vi "log_error.vi"(6 "timestamp":timestamp, 7 "context":string, 8 "error in (no error)":errorcluster, 9 "level":T1=200 items=["OFF"=0, "FATAL"=100, "ERROR"=200, "WARN"=300, "INFO"=400, "DEBUG"=500, "TRACE"=600, "ALL"=65535], 11 "Queue Log Provider in":refnum<class "NIErrLog Log Provider.lvclass">) -> (0 "error out":errorcluster, 3 "Queue Log Provider out":refnum<class "NIErrLog Log Provider.lvclass">)   [LabVIEW 2019, in "LVCOOOP.lvlib" / "Support API.lvlib" / "NIErrLog Log Provider.lvclass"]
uses:
  NIErrLog Log Provider.lvclass
  Log Service/public/level.ctl
  Log Service/Log Service.lvclass
  <vilib>/Utility/SystemLogging/NI_SystemLogging.lvlib
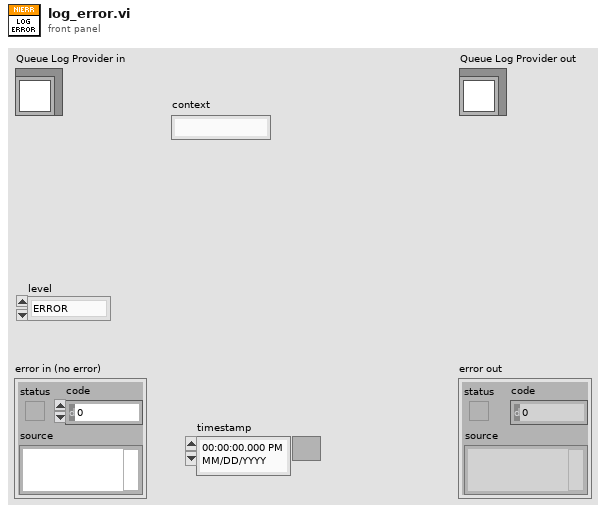
[diagram p1: front panel]
types:
  T1 = typedef "LVCOOOP.lvlib/Support API.lvlib/Log Service.lvclass/level.ctl" = u16
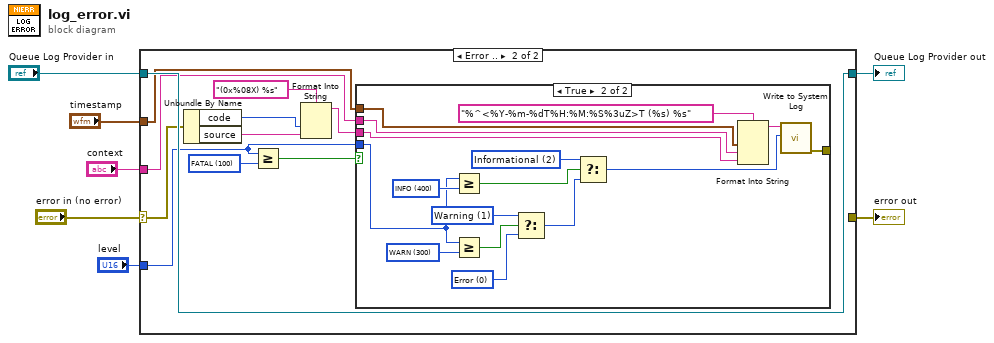
[diagram p0: block diagram]
diagram:
  n1 = case shown="Error .." "error in (no error)" {
    selector: "error in (no error)" -> [w9 w19]
    tunnel: [w9 _] -> w1
    tunnel: "timestamp" -> [_ w13]
    tunnel: "level" -> [_ w10]
    tunnel: "context" -> [_ w12]
    tunnel: [w8 w20] -> w5
    tunnel: "Queue Log Provider in" -> [w8 w20]
    frame No Error {
    }
    frame Error {
      w15 = T1 100 items=["OFF"=0, "FATAL"=100, "ERROR"=200, "WARN"=300, "INFO"=400, "DEBUG"=500, "TRACE"=600, "ALL"=65535] ("level")
      n2 = Unbundle By Name(w19) -> ("code"=w17:i32, "source"=w16:string)
      n3 = Greater Or Equal?(x=w10, y=w15) -> (x >= y?=w14:bool)
      n4 = Format Into String(format string="(0x%08X) %s", w17, w16) -> (resulting string=w11:string)  [unwired: 2 in, 1 out]
      n5 = case shown="True" w14 {
        tunnel: w10 -> [_ w29]
        tunnel: [_ w26] -> _
        tunnel: w11 -> [_ w21]
        tunnel: w12 -> [_ w22]
        tunnel: w13 -> [_ w23]
        frame False {
        }
        frame True {
          w28 = 0 items=["Error", "Warning", "Informational"] ("severity")
          w31 = 1 items=["Error", "Warning", "Informational"] ("severity")
          w33 = T1 300 items=["OFF"=0, "FATAL"=100, "ERROR"=200, "WARN"=300, "INFO"=400, "DEBUG"=500, "TRACE"=600, "ALL"=65535] ("level")
          w34 = 2 items=["Error", "Warning", "Informational"] ("severity")
          w36 = T1 400 items=["OFF"=0, "FATAL"=100, "ERROR"=200, "WARN"=300, "INFO"=400, "DEBUG"=500, "TRACE"=600, "ALL"=65535] ("level")
          n6 = Greater Or Equal?(x=w29, y=w36) -> (x >= y?=w35:bool)
          n7 = Greater Or Equal?(x=w29, y=w33) -> (x >= y?=w32:bool)
          n8 = Select(t=w31, s=w32, f=w28) -> (s? t:f=w30:i32)
          n9 = Select(t=w34, s=w35, f=w30) -> (s? t:f=w27:i32)
          n10 = Format Into String(format string="%^<%Y-%m-%dT%H:%M:%S%3uZ>T (%s) %s", w23, w22, w21) -> (resulting string=w24:string)  [unwired: 2 in, 1 out]
          n11 = call <vilib>:"Write to System Log.vi"("severity"=w27, "message"=w24) -> ("error out"=w26:errorcluster)  [unwired: 9 in]
        }
      }
    }
  }
  "error out" <- w1
  "Queue Log Provider out" <- w5
